vi "agilent_34970A_resistances.vi"(5 "Agilent 34970A Port":refnum<visa-resource-name>="COM35", 6 "Channels":string="101,102,103,104", 7 "Readings":u16=1) -> (0 "Avg R1":dbl=nan format="%_6f", 1 "Avg R2":dbl=nan format="%_6f", 2 "Avg R3":dbl=nan format="%_6f", 3 "Avg R4":dbl=nan format="%_6f", 4 "Resistances":string)   [LabVIEW 2010]
uses:
  <vilib>/Analysis/NI_AALBase.lvlib
panel:
  out "Std Dev R4":dbl=-0.0 format="%_6f"
  out "R4 Array":dbl[](array[numeric])
  out "Std Dev R3":dbl=-0.0 format="%_6f"
  out "R3 Array":dbl[](array[numeric])
  out "Std Dev R2":dbl=-0.0 format="%_6f"
  out "R2 Array":dbl[](array[numeric])
  out "R1 Array":dbl[](array[numeric])
  out "Std Dev R1":dbl=-0.0 format="%_6f"
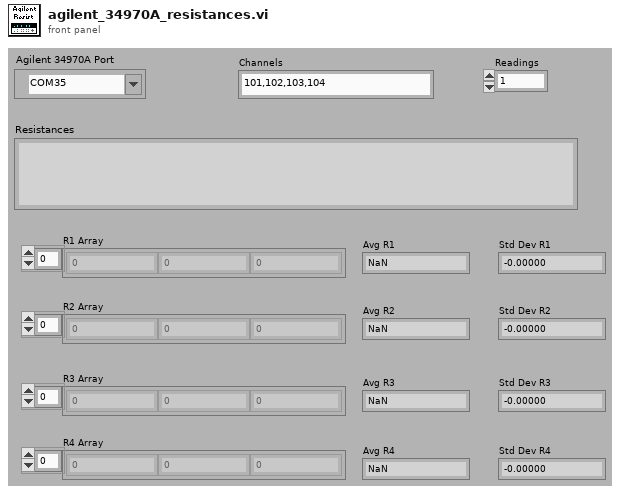
[diagram p1: front panel]
types:
  T1 = enum16{"Enable Register", "Event Register", "Operation Complete Bit"}
  T2 = enum16{"Manual", "Minimum", "Maximum", "Infinity"}
  T3 = enum16{"Bus", "Immediate", "External", "Alarm 1", "Alarm 2", "Alarm 3", "Alarm 4", "Timer"}
  T4 = cluster{"Include Alarm Data? (F:No)":bool, "Include Channel #? (F:No)":bool, "Include Time? (F:No)":bool, "Include Units? (F:No)":bool}
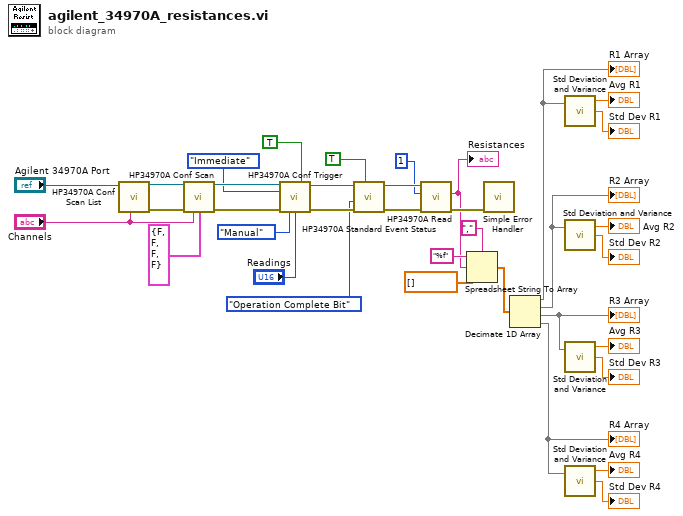
[diagram p0: block diagram]
diagram:
  n1 = call "HP34970A Conf Scan List.vi"("Scan List (empty)"="Channels", "VISA resource name"="Agilent 34970A Port") -> ("error out"=w32:errorcluster, "VISA resource name out"=w33:refnum<visa-resource-name>)  [unwired: 7 in, 1 out]
  n2 = call "HP34970A Conf Scan.vi"("VISA resource name"=w33, "error in (no error)"=w32, "Channel List (empty)"="Channels", "Scan Fields"=T4 {"Include Alarm Data? (F:No)"=FALSE, "Include Channel #? (F:No)"=FALSE, "Include Time? (F:No)"=FALSE, "Include Units? (F:No)"=FALSE}) -> ("VISA resource name out"=w30:refnum<visa-resource-name>, "error out"=w29:errorcluster)  [unwired: 9 in, 1 out]
  n3 = call "HP34970A Conf Trigger.vi"("VISA resource name"=w30, "Wait for Trigger? (F:No)"=TRUE, "Source (1:Immediate)"=T3."Immediate", "error in (no error)"=w29, "Max Trigger Count (3:Inf)"=T2."Manual", "# Triggers (1)"="Readings") -> ("VISA resource name out"=w24:refnum<visa-resource-name>, "error out"=w23:errorcluster)  [unwired: 7 in, 1 out]
  n4 = call "HP34970A Standard Event Status.vi"("Set/Check? (F:Set)"=TRUE, "error in (no error)"=w23, "Check Parameter (0:Enable Reg)"=T1."Operation Complete Bit", "VISA resource name"=w24) -> ("error out"=w35:errorcluster, "VISA resource name out"=w34:refnum<visa-resource-name>)  [unwired: 5 in, 1 out]
  n5 = call "HP34970A Read.vi"("error in (no error)"=w35, "# Channels (1)"=1, "VISA resource name"=w34) -> ("error out"=w36:errorcluster, "Readings"=w12:string)  [unwired: 5 in, 2 out]
  "Resistances" <- w12
  n6 = Spreadsheet String To Array(delimiter (Tab)=",", format string="%f", spreadsheet string=w12, array type (2D Dbl)=dbl[] []) -> (array=w11:dbl[])
  n7 = call <vilib>:"Simple Error Handler.vi"("error in (no error)"=w36) -> ()  [unwired: 4 in, 5 out]
  n8 = Decimate 1D Array(w11) -> (w10:dbl[], w3:dbl[], w2:dbl[], w1:dbl[])
  "R1 Array" <- w10
  "R2 Array" <- w3
  "R3 Array" <- w2
  "R4 Array" <- w1
  n9 = call <vilib>:"Std Deviation and Variance.vi"("X"=w10) -> ("mean"=→"Avg R1":dbl, "standard deviation"=→"Std Dev R1":dbl)  [unwired: 1 in, 1 out]
  n10 = call <vilib>:"Std Deviation and Variance.vi"("X"=w3) -> ("mean"=→"Avg R2":dbl, "standard deviation"=→"Std Dev R2":dbl)  [unwired: 1 in, 1 out]
  n11 = call <vilib>:"Std Deviation and Variance.vi"("X"=w2) -> ("mean"=→"Avg R3":dbl, "standard deviation"=→"Std Dev R3":dbl)  [unwired: 1 in, 1 out]
  n12 = call <vilib>:"Std Deviation and Variance.vi"("X"=w1) -> ("mean"=→"Avg R4":dbl, "standard deviation"=→"Std Dev R4":dbl)  [unwired: 1 in, 1 out]
